vi "DSF.Engine.Timing.Set Offset.vi"(10 "Offset":u64, 11 "Timing in":refnum<class "DSF.Engine.Timing.lvclass">) -> (3 "Timing out":refnum<class "DSF.Engine.Timing.lvclass">)   [LabVIEW 2017, in "Data Sharing Framework Engine.lvlib" / "DSF.Engine.Timing.lvclass"]
uses:
  DSF.Engine.Timing.lvclass
  DSF.Engine.Timing.lvclass/DSF.Engine.Timing.ctl
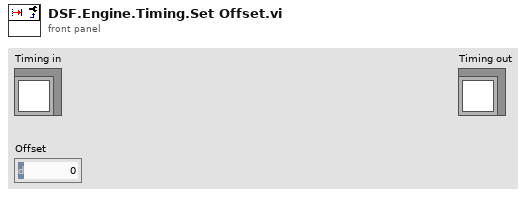
[diagram p1: front panel]
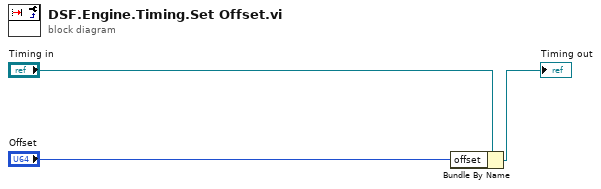
[diagram p0: block diagram]
diagram:
  n1 = Bundle By Name(cluster="Timing in", "offset"="Offset") -> (→"Timing out":refnum<class "DSF.Engine.Timing.lvclass">)
